vi "Post action.vi"(6 "Index":i32=41, 8 "error in (no error)":errorcluster, 9 "PostAction":T1, 11 "SweepControl":refnum<class "Sweep Control.lvclass">) -> (0 "error out":errorcluster, 3 "SweepControl":refnum<class "Sweep Control.lvclass">)   [LabVIEW 2019, in "Sweep Control.lvclass"]
uses:
  Sweep Control.lvclass
  Typedefs/Enum - PostAction.ctl
  Sweep Control.lvclass/Sweep Control.ctl
  <userlib>/LevyLab/Transport/Transport/Transport.lvclass/Transport.ctl
  <userlib>/LevyLab/Transport/Control Experiment/Control Experiment.lvclass/Control Experiment.ctl
  <userlib>/LevyLab/Transport/Transport/Transport.lvclass
  <userlib>/LevyLab/Transport/Control Experiment/Control Experiment.lvclass
  <userlib>/LevyLab/Instrument Framework/Instrument Types/Cryostat/Instrument.Cryostat.lvclass
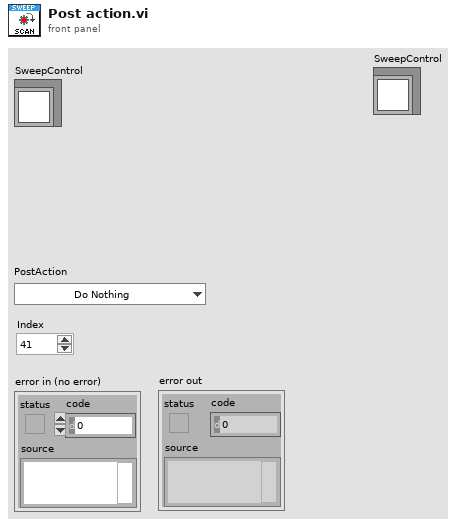
[diagram p1: front panel]
types:
  T1 = typedef "Sweep Control.lvclass/Enum - PostAction.ctl" = enum16{"Do Nothing", "Wait (time)", "Wait (Temperature)", "Wait (<T ; B sweep)", "Wait (Magnet)"}
  T2 = typedef "Sweep Control.lvclass/Cluster - ScanParamters.ctl" = cluster{"Start":dbl, "End":dbl, "Step":dbl, "Rate":dbl, "Waveform type":enum16{"linear", "triangle", "power"}, "wait (ms or K)":dbl, "Address":string, "channel":i32}
  T3 = typedef "Control Experiment.lvclass/Instrument Classes--cluster.ctl" = cluster{"DAQ":refnum<class "Instrument.LockinAPI.lvclass">, "Amplifier":refnum<class "Instrument.Amplifier.lvclass">, "Temperature":refnum<class "Instrument.Cryostat.lvclass">, "Magnet":refnum<class "Instrument.Cryostat.lvclass">, "Rotator":refnum<class "Instrument.Cryostat.lvclass">, "Level":refnum<class "Instrument.Cryostat.lvclass">, "Capacitance":refnum<class "Instrument.CBridge.lvclass">, "Delay Line":refnum<class "Instrument.DelayLine.lvclass">, "Strain Cell":refnum<class "Instrument.Strain.lvclass">, "VNA":refnum<class "Instrument.VNA.lvclass">, "Source":refnum<class "Instrument.VSource.lvclass">}
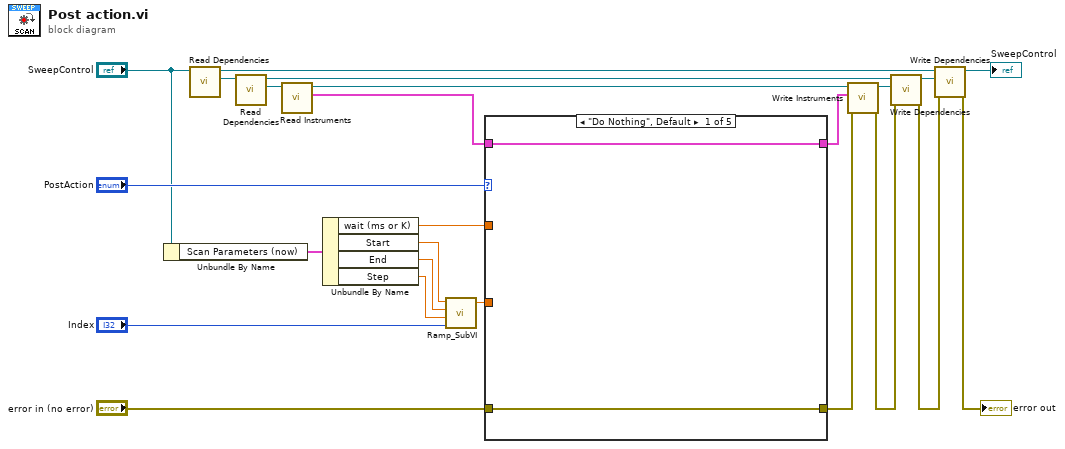
[diagram p0: block diagram]
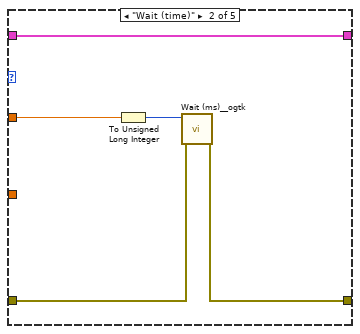
[diagram p2: hidden frame]
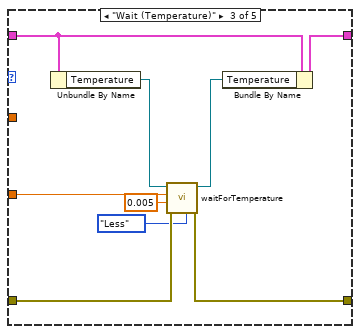
[diagram p3: hidden frame]
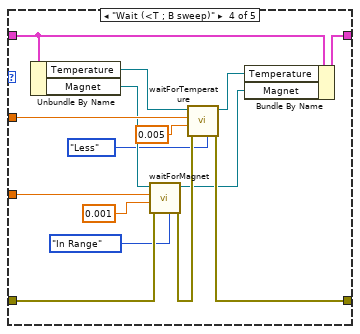
[diagram p4: hidden frame]
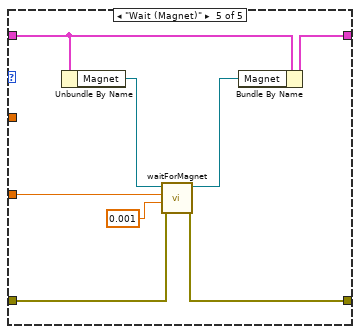
[diagram p5: hidden frame]
diagram:
  n1 = Unbundle By Name("SweepControl") -> ("Scan Parameters (now)"=w17:T2)
  n2 = call <userlib>:"Read Dependencies.vi"("SweepControl in"="SweepControl") -> ("Transport"=w11:refnum<class "Transport.lvclass">, "SweepControl out"=w4:refnum<class "Sweep Control.lvclass">)  [unwired: 8 in, 1 out]
  n3 = call <userlib>:"Read Dependencies.vi"("Transport"=w11) -> ("C.E."=w12:refnum<class "Control Experiment.lvclass">, "Transport"=w6:refnum<class "Transport.lvclass">)  [unwired: 8 in, 1 out]
  n4 = call <userlib>:"Read Instruments.vi"("Control Experiment in"=w12) -> ("Instruments"=w1:T3, "Control Experiment out"=w5:refnum<class "Control Experiment.lvclass">)  [unwired: 8 in, 1 out]
  n5 = Unbundle By Name(w17) -> ("wait (ms or K)"=w18:dbl, "Start"=w21:dbl, "End"=w20:dbl, "Step"=w19:dbl)
  n6 = call <userlib>:"Ramp_SubVI.vi"("index"="Index", "step"=w19, "end"=w20, "start"=w21) -> ("Numeric"=w23:dbl)  [unwired: 1 in, 1 out]
  n7 = case shown="\"Do Nothing\", Default" "PostAction" {
    tunnel: w23 -> [_ _ w40 w53 w63]
    tunnel: w18 -> [_ w31 _ w54 _]
    tunnel: "error in (no error)" -> [w26 w30 w39 w52 w62]
    tunnel: [w26 w29 w38 w55 w61] -> w14
    tunnel: w1 -> [w25 w27 w36 w49 w59]
    tunnel: [w25 w27 w34 w47 w57] -> w15
    frame "Do Nothing", Default {
    }
    frame "Wait (time)" {
      n8 = To Unsigned Long Integer(number=w31) -> (unsigned 32bit integer=w28:u32)
      n9 = call <userlib>:"Wait (ms)__ogtk.vi"("error in (no error)"=w30, "milliseconds to wait"=w28) -> ("error out"=w29:errorcluster)  [unwired: 8 in, 1 out]
    }
    frame "Wait (Temperature)" {
      n10 = Unbundle By Name(w36) -> ("Temperature"=w37:refnum<class "Instrument.Cryostat.lvclass">)
      n11 = call <userlib>:"waitForTemperature.vi"("Type"=enum16{"In Range", "Less", "Greater"}."Less", "error in (no error)"=w39, "Tolerance (K)"=0.005, "Setpoint (K)"=w40, "Instrument.Cryostat in"=w37) -> ("error out"=w38:errorcluster, "Instrument.Cryostat out"=w35:refnum<class "Instrument.Cryostat.lvclass">)  [unwired: 5 in]
      n12 = Bundle By Name(cluster=w36, "Temperature"=w35) -> (w34:T3)
    }
    frame "Wait (<T ; B sweep)" {
      n13 = Unbundle By Name(w49) -> ("Temperature"=w45:refnum<class "Instrument.Cryostat.lvclass">, "Magnet"=w50:refnum<class "Instrument.Cryostat.lvclass">)
      n14 = call <userlib>:"waitForMagnet.vi"("Type"=enum16{"In Range", "Less", "Greater"}."In Range", "error in (no error)"=w52, "Tolerance (T)"=0.001, "Setpoint (T)"=w53, "Instrument.Cryostat in"=w50) -> ("error out"=w51:errorcluster, "Instrument.Cryostat out"=w48:refnum<class "Instrument.Cryostat.lvclass">)  [unwired: 5 in]
      n15 = call <userlib>:"waitForTemperature.vi"("Type"=enum16{"In Range", "Less", "Greater"}."Less", "error in (no error)"=w51, "Tolerance (K)"=0.005, "Setpoint (K)"=w54, "Instrument.Cryostat in"=w45) -> ("error out"=w55:errorcluster, "Instrument.Cryostat out"=w46:refnum<class "Instrument.Cryostat.lvclass">)  [unwired: 5 in]
      n16 = Bundle By Name(cluster=w49, "Temperature"=w46, "Magnet"=w48) -> (w47:T3)
    }
    frame "Wait (Magnet)" {
      n17 = Unbundle By Name(w59) -> ("Magnet"=w60:refnum<class "Instrument.Cryostat.lvclass">)
      n18 = call <userlib>:"waitForMagnet.vi"("error in (no error)"=w62, "Tolerance (T)"=0.001, "Setpoint (T)"=w63, "Instrument.Cryostat in"=w60) -> ("error out"=w61:errorcluster, "Instrument.Cryostat out"=w58:refnum<class "Instrument.Cryostat.lvclass">)  [unwired: 6 in]
      n19 = Bundle By Name(cluster=w59, "Magnet"=w58) -> (w57:T3)
    }
  }
  n20 = call <userlib>:"Write Instruments.vi"("error in (no error)"=w14, "Instruments"=w15, "Control Experiment in"=w5) -> ("error out"=w13:errorcluster, "Control Experiment out"=w16:refnum<class "Control Experiment.lvclass">)  [unwired: 7 in]
  n21 = call <userlib>:"Write Dependencies.vi"("error in (no error)"=w13, "Control Experiment"=w16, "Transport in"=w6) -> ("error out"=w8:errorcluster, "Transport out"=w10:refnum<class "Transport.lvclass">)  [unwired: 7 in]
  n22 = call <userlib>:"Write Dependencies.vi"("error in (no error)"=w8, "Transport"=w10, "SweepControl in"=w4) -> ("error out"=→"error out":errorcluster, "SweepControl out"=→"SweepControl":refnum<class "Sweep Control.lvclass">)  [unwired: 7 in]
